vi "Populate gRPC Events.vi"(7 "RPC Method Parameters":T1[](array[typedef]), 8 "error in (no error)":errorcluster, 10 "Server class in":refnum<vi>, 11 "Server library in":refnum<vi>) -> (0 "error out":errorcluster, 2 "Server class out":refnum<vi>, 3 "Server library out":refnum<vi>)   [LabVIEW 2019, in "gRPC Scripting Tools.lvlib"]
uses:
  gRPC Scripting Tools.lvlib
  TypeDefs/RPC Method Parameters.ctl
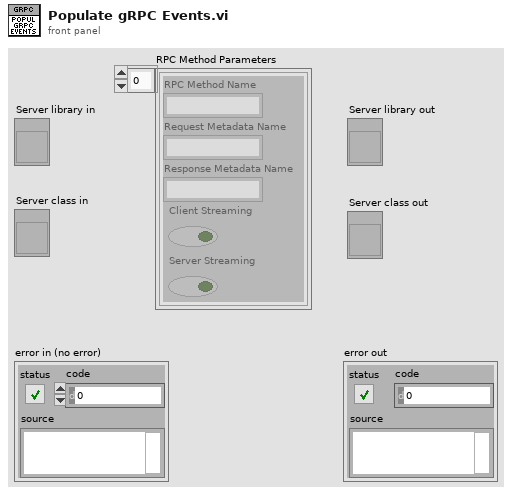
[diagram p1: front panel]
types:
  T1 = typedef "gRPC Scripting Tools.lvlib/RPC Method Parameters.ctl" = cluster{"RPC Method Name":string, "Request Metadata Name":string, "Response Metadata Name":string, "Client Streaming":bool, "Server Streaming":bool}
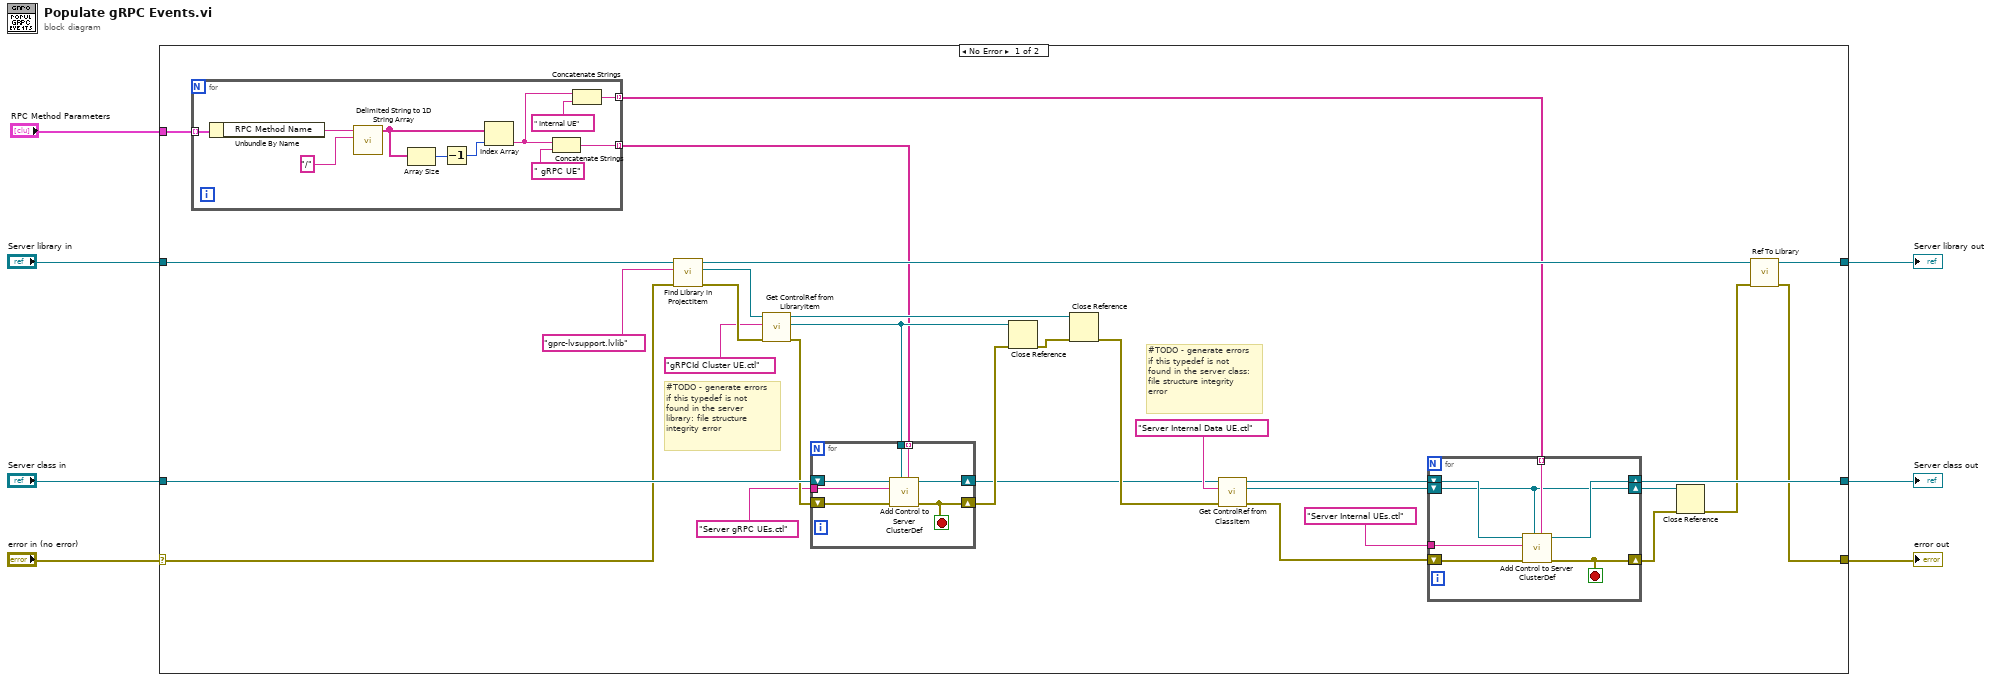
[diagram p0: block diagram]
diagram:
  n1 = case shown="No Error" "error in (no error)" {
    selector: "error in (no error)" -> [w17 w63]
    tunnel: [w14 w63] -> w7
    tunnel: [w37 w65] -> w6
    tunnel: [w15 w64] -> w2
    tunnel: "Server class in" -> [w35 w65]
    tunnel: "Server library in" -> [w34 w64]
    tunnel: "RPC Method Parameters" -> [w13 _]
    frame No Error {
      # "#TODO - generate errors if this typedef is not found in the server library: file structure integrity error"
      # "#TODO - generate errors if this typedef is not found in the server class: file structure integrity error"
      n2 = for {
        tunnel: w13 -> [w43] mode=indexing
        tunnel: [w41] -> w12 mode=indexing
        tunnel: [w38] -> w11 mode=indexing
        n3 = Unbundle By Name(w43) -> ("RPC Method Name"=w47:string)
        n4 = call <vilib>:"Delimited String to 1D String Array.vi"("delimiter"="/", "delimited string"=w47) -> ("string array"=w44:string[])  [unwired: 9 in]
        n5 = Array Size(array=w44) -> (size(s)=w46:i32)
        n6 = Decrement(x=w46) -> (x-1=w45:i32)
        n7 = Index Array(array=w44, index=w45) -> (element=w40:string)
        n8 = Concatenate Strings(w40, " gRPC UE" ("string")) -> (w41:string)
        n9 = Concatenate Strings(w40, " Internal UE" ("string")) -> (w38:string)
      }
      n10 = call "Find Library in ProjectItem.vi"("error in (no error)"=w17, "Library Name"="gprc-lvsupport.lvlib", "ProjectItem in"=w34) -> ("error out"=w22:errorcluster, "Library out"=w19:refnum<vi>, "ProjectItem out"=w16:refnum<vi>)  [unwired: 5 in, 1 out]
      n11 = call "Get ControlRef from LibraryItem.vi"("error in (no error)"=w22, "Control Name"="gRPCId Cluster UE.ctl" ("y"), "Library item in"=w19) -> ("error out"=w33:errorcluster, "Control ref out"=w30:refnum<vi>, "Library item out"=w32:refnum<vi>)  [unwired: 5 in, 1 out]
      n12 = for {
        tunnel: "Server gRPC UEs.ctl" ("Item Name") -> [w60]
        tunnel: w30 -> [w59]
        shift-right: [w56] -> w29
        shift-left: w33 -> [w62]
        tunnel: w12 -> [w58] mode=indexing
        shift-right: [w57] -> w24
        shift-left: w35 -> [w61]
        stop <- w56 stop-if-true
        n13 = call "Add Control to Server ClusterDef.vi"("New Control Label"=w58, "Source Control ref in"=w59, "error in (no error)"=w62, "Target ClusterDef Name"=w60, "Server class in"=w61) -> ("error out"=w56:errorcluster, "Server class out"=w57:refnum<vi>)  [unwired: 5 in]
      }
      n14 = Close Reference(reference=w30, error in (no error)=w29) -> (error out=w31:errorcluster)
      n15 = Close Reference(reference=w32, error in (no error)=w31) -> (error out=w36:errorcluster)
      n16 = call "Get ControlRef from ClassItem.vi"("error in (no error)"=w36, "Item Name"="Server Internal Data UE.ctl", "LVClassLibrary in"=w24) -> ("error out"=w27:errorcluster, "Control ref out"=w28:refnum<vi>, "LVClassLibrary out"=w26:refnum<vi>)  [unwired: 5 in, 1 out]
      n17 = for {
        tunnel: "Server Internal UEs.ctl" ("Target ClusterDef Name") -> [w53]
        tunnel: w11 -> [w52] mode=indexing
        shift-right: [w51] -> w37
        shift-left: w26 -> [w54]
        shift-right: [w50] -> w10
        shift-left: w27 -> [w55]
        shift-right: [w49] -> w9
        shift-left: w28 -> [w49]
        stop <- w50 stop-if-true
        n18 = call "Add Control to Server ClusterDef.vi"("New Control Label"=w52, "Source Control ref in"=w49, "error in (no error)"=w55, "Target ClusterDef Name"=w53, "Server class in"=w54) -> ("error out"=w50:errorcluster, "Server class out"=w51:refnum<vi>)  [unwired: 5 in]
      }
      n19 = Close Reference(reference=w9, error in (no error)=w10) -> (error out=w8:errorcluster)
      n20 = call "Ref To Library.vi"("error in (no error)"=w8, "ProjectItem in"=w16) -> ("error out"=w14:errorcluster, "Library out"=w15:refnum<vi>)  [unwired: 8 in]
    }
    frame Error {
    }
  }
  "error out" <- w7
  "Server class out" <- w6
  "Server library out" <- w2
